vi "LUCS001RT_GPS_RS232_ReceiverFIFO.vi"(0 "error in":errorcluster, 1 "RxArrayIn":u8[](array[numeric])=[0, 0, 0, 0, 0, 0, 0, 0, 0, 0, 0, 0, 0, 0, 0, 0, 0, 0, 0, 0, 0, 0, 0, 0, 0, 0, 0, 0, 0, 0, 0, 0, 0, 0, 0, 0, 0, 0, 0, 0, 0, 0, 0, 0, 0, 0, 0, 0, 0, 0, 0, 0, 0, 0, 0, 0, 0, 0, 0, 0, 0, 0, 0, 0, 0, 0, 0, 0, 0, 0, 0, 0, 0, 0, 0, 0, 0, 0, 0, 0, 0, 0, 0, 0, 0, 0, 0, 0, 0, 0, 0, 0, 0, 0, 0, 0, 0, 0, 0, 0] format="%.0x", 5 "TimedOut":bool, 9 "CurrentLoopIndex":i32, 11 "FIFODataIn":u32[](array[numeric]) format="%02x", 12 "UpdateStateIn":bool, 13 "MarkIndexIn":i32 format="%08x") -> (3 "RxArrayOut":u8[](array[numeric]) format="%.0x", 4 "error out":errorcluster, 10 "DataReady":bool, 14 "MarkIndexOut":i32 format="%08x", 15 "UpdateStateOut":bool)   [LabVIEW 2020]
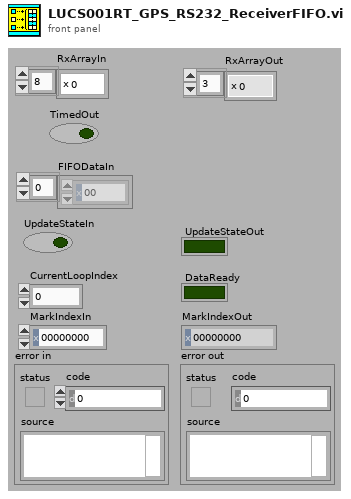
[diagram p1: front panel]
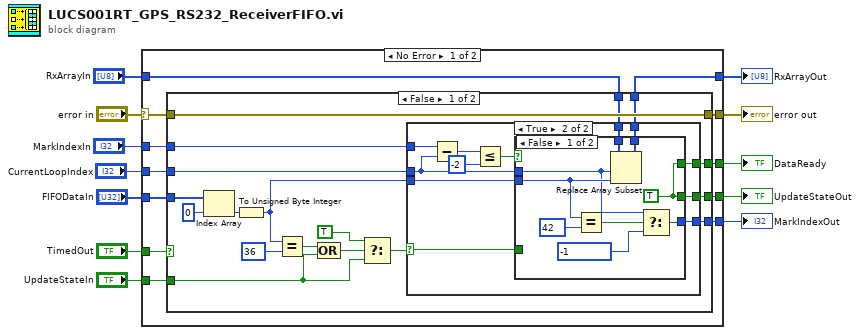
[diagram p0: block diagram]
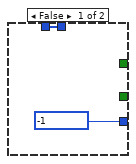
[diagram p2: hidden frame]
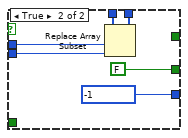
[diagram p3: hidden frame]
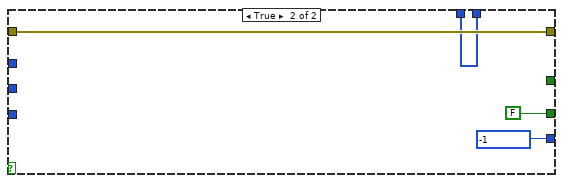
[diagram p4: hidden frame]
diagram:
  n1 = case shown="No Error" "error in" {
    selector: "error in" -> [w17 w76]
    tunnel: [w24 _] -> w12
    tunnel: "UpdateStateIn" -> [w23 _]
    tunnel: "TimedOut" -> [w22 _]
    tunnel: [w21 _] -> w5
    tunnel: "RxArrayIn" -> [w20 _]
    tunnel: "FIFODataIn" -> [w19 _]
    tunnel: [w18 w76] -> w8
    tunnel: "CurrentLoopIndex" -> [w16 _]
    tunnel: [w15 _] -> w3
    tunnel: "MarkIndexIn" -> [w14 _]
    tunnel: [w13 _] -> w1
    frame No Error {
      n2 = case shown="False" w22 {
        tunnel: w17 -> [w42 w75]
        tunnel: [w42 w75] -> w18
        tunnel: w19 -> [w39 _]
        tunnel: w20 -> [w41 w73]
        tunnel: [w40 w73] -> w21
        tunnel: w23 -> [w28 _]
        tunnel: [w30 FALSE] -> w24
        tunnel: w16 -> [w29 _]
        tunnel: [w27 -1 ("f")] -> w15
        tunnel: w14 -> [w26 _]
        tunnel: [w25 _] -> w13
        frame False {
          n3 = Index Array(array=w39, index=0) -> (element=w38:u32)
          n4 = To Unsigned Byte Integer(number=w38) -> (unsigned 8bit integer=w36:u8)
          n5 = Equal?(x=w36, y=u8 36) -> (x = y?=w34:bool)
          n6 = Compound Arithmetic op=OR(w34, w28) -> (w32:bool)
          n7 = Select(t=TRUE, s=w32, f=w28) -> (s? t:f=w31:bool)
          n8 = case shown="True" w31 {
            selector: w31 -> [_ w54]
            tunnel: w41 -> [w44 w56]
            tunnel: [w44 w55] -> w40
            tunnel: w36 -> [_ w52]
            tunnel: [_ w53] -> w30
            tunnel: w29 -> [_ w49]
            tunnel: [-1 ("f") w51] -> w27
            tunnel: w26 -> [_ w50]
            tunnel: [_ w45] -> w25
            frame False {
            }
            frame True {
              n9 = Subtract(x=w50, y=w49) -> (x-y=w48:i32)
              n10 = Less Or Equal?(x=w48, y=-2) -> (x <= y?=w46:bool)
              n11 = case shown="False" w46 {
                tunnel: w56 -> [w65 w71]
                tunnel: [w64 w70] -> w55
                tunnel: w54 -> [_ _]
                tunnel: [w57 FALSE ("t")] -> w53
                tunnel: w52 -> [w62 w69]
                tunnel: w49 -> [w60 w67]
                tunnel: [w58 -1 ("f")] -> w51
                tunnel: [w57 _] -> w45
                frame False {
                  w57 = TRUE ("t")
                  n12 = Equal?(x=w62, y=u8 42) -> (x = y?=w61:bool)
                  n13 = Replace Array Subset(array=w65, new element=w62, index=w60) -> (w64:u8[])
                  n14 = Select(t=w60, s=w61, f=-1) -> (s? t:f=w58:i32)
                }
                frame True {
                  n15 = Replace Array Subset(array=w71, new element=w69, index=w67) -> (w70:u8[])
                }
              }
            }
          }
        }
        frame True {
        }
      }
    }
    frame Error {
    }
  }
  "UpdateStateOut" <- w12
  "error out" <- w8
  "RxArrayOut" <- w5
  "MarkIndexOut" <- w3
  "DataReady" <- w1
